vi "cmd1.vi"() -> ()   [LabVIEW 2010]
panel:
  out "reversed":string
  in  "Param":variant
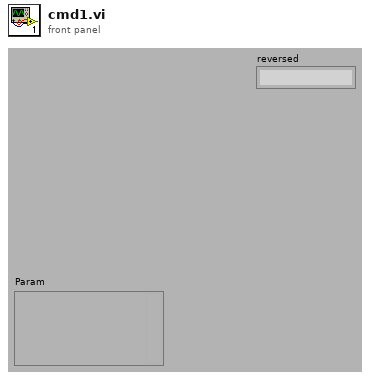
[diagram p1: front panel]
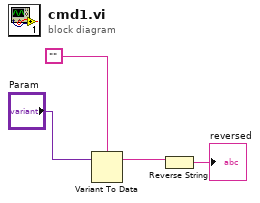
[diagram p0: block diagram]
diagram:
  n1 = Variant To Data(Variant="Param", type="") -> (data=w2:string)  [unwired: 1 in, 1 out]
  n2 = Reverse String(1:w2) -> (0:→"reversed":string)
